vi "test.vi"(8 "error in (no error)":errorcluster, 11 "Class 2 in":refnum<class "Class 2.lvclass">) -> (0 "error out":errorcluster, 3 "Class 2 out":refnum<class "Class 2.lvclass">)   [LabVIEW 2023, in "Class 2.lvclass"]
uses:
  Class 2.lvclass
  Class 2.lvclass/Class 2.ctl
  class1/Class 1.lvclass
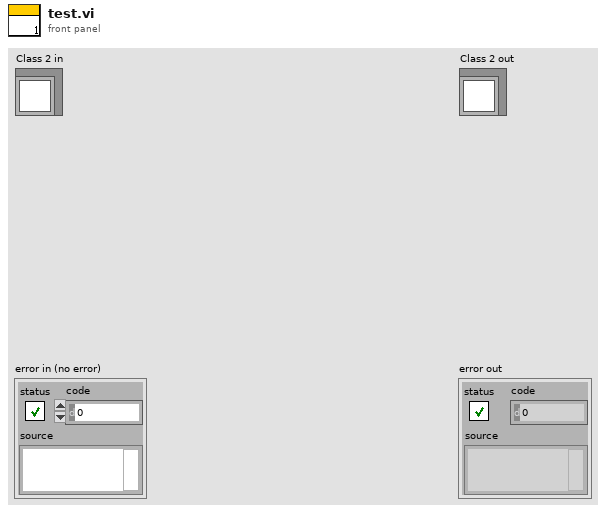
[diagram p1: front panel]
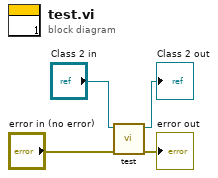
[diagram p0: block diagram]
diagram:
  n1 = call-parent "test.vi"("error in (no error)"="error in (no error)", "Class 1 in"="Class 2 in") -> ("error out"=→"error out":errorcluster, "Class 1 out"=→"Class 2 out":refnum<class "Class 2.lvclass">)  [unwired: 8 in]
